vi "Get Rx Timestamp Data Channel Reference.vi"(8 "error in":errorcluster, 11 "frame ref in":T1 format="%.0x") -> (0 "error out":errorcluster, 2 "timestamp channel data reference":T2 format="%.0x", 3 "frame ref out":T1 format="%.0x", 4 "timestamp channel found?":bool)   [LabVIEW 2020]
uses:
  <vilib>/NI VeriStand/Custom Device Tools/Custom Device Utility Library/Custom Device Utility Library.lvlib
  <vilib>/NI VeriStand/Custom Device API/Data Access Type.ctl
  <vilib>/NI VeriStand/Custom Device API/Custom Device API.lvlib
  Scripting/Constants.vi
  Scripting/Ballard ARINC 429 Scripting.lvlib
  <vilib>/NI VeriStand/Custom Device Tools/Custom Device Utility Library/NI VeriStand - Search for Item by GUID.vi
  <vilib>/NI VeriStand/Custom Device API/Custom Device Item Ref.ctl
  <vilib>/NI VeriStand/Custom Device API/Data Reference.ctl
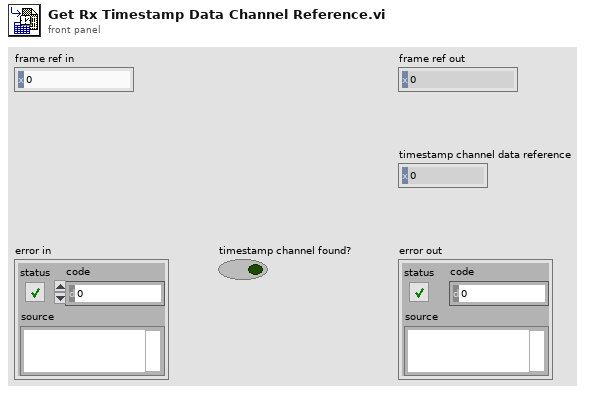
[diagram p1: front panel]
types:
  T1 = typedef "Custom Device API.lvlib/Custom Device Item Ref.ctl" = u64
  T2 = typedef "Custom Device API.lvlib/Data Reference.ctl" = i32
  T3 = typedef "Custom Device API.lvlib/Data Access Type.ctl" = enum16{"Read", "Write"}
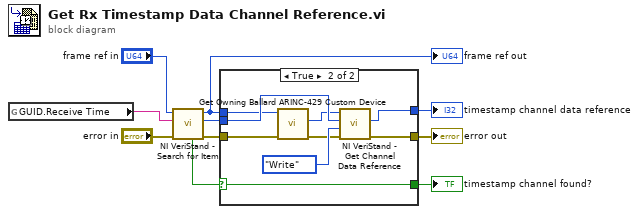
[diagram p0: block diagram]
diagram:
  n1 = global read "Constants.vi" "GUID.Receive Time"() -> (w10:string)
  n2 = call-poly <vilib>:"NI VeriStand - Search for Item.vi"("error in"="error in", "Item GUID"=w10, "Section Ref in"="frame ref in") -> ("error out"=w2:errorcluster, "Item Ref"=w3:T1, "Section Ref out"=w1:T1, "Found"=w8:bool)  [unwired: 5 in]
  "frame ref out" <- w1
  n3 = case shown="True" w8 {
    selector: w8 -> [w11 w17]
    tunnel: w3 -> [_ w20]
    tunnel: [_ w19] -> w6
    tunnel: w2 -> [w12 w14]
    tunnel: [w12 w18] -> w7
    tunnel: [w11 w17] -> w9
    tunnel: w1 -> [_ w16]
    frame False {
    }
    frame True {
      n4 = call "Get Owning Ballard ARINC-429 Custom Device.vi"("error in"=w14, "item ref in"=w16) -> ("error out"=w15:errorcluster, "owning Ballard ARINC-429 custom device"=w13:T1)  [unwired: 7 in, 1 out]
      n5 = call <vilib>:"NI VeriStand - Get Channel Data Reference.vi"("error in (no error)"=w15, "Access"=Data_Access_Type."Write", "Channel Ref in"=w20, "Device Ref in"=w13) -> ("error out"=w18:errorcluster, "Channel Data Reference"=w19:T2)  [unwired: 5 in, 1 out]
    }
  }
  "timestamp channel found?" <- w9
  "error out" <- w7
  "timestamp channel data reference" <- w6
